vi "Read PathControl.lvclass.vi"(11 "Test Framework in":refnum<class "Test Framework.lvclass">) -> (2 "PathControl.lvclass":refnum<class "PathControl.lvclass">, 3 "Test Framework out":refnum<class "Test Framework.lvclass">)   [LabVIEW 2020, in "Test Framework.lvclass"]
uses:
  Test Framework.lvclass
  Path Control/PathControl.lvclass
  Test Framework.lvclass/Test Framework.ctl
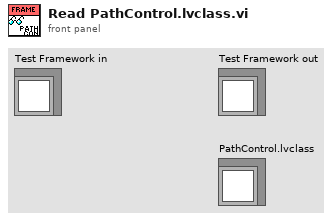
[diagram p1: front panel]
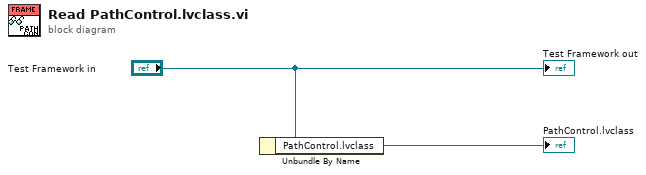
[diagram p0: block diagram]
diagram:
  n1 = Unbundle By Name("Test Framework in") -> ("PathControl.lvclass"=→"PathControl.lvclass":refnum<class "PathControl.lvclass">)
  "Test Framework out" <- "Test Framework in"
